vi "Get Panther Dashboard Version.vi"() -> (3 "Panther Dashboard Version":string)   [LabVIEW 2019, in "Panther Dashboard.lvlib"]
uses:
  Panther Dashboard.lvlib
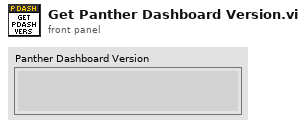
[diagram p1: front panel]
types:
  T1 = cluster{"Major":u16, "Minor":u16, "Fix":u16, "Build":u16}
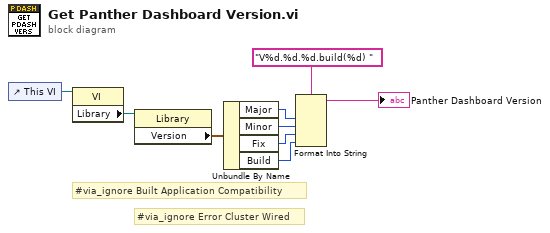
[diagram p0: block diagram]
diagram:
  # "#via_ignore Built Application Compatibility"
  # "#via_ignore Error Cluster Wired"
  n1 = control-ref of="This VI"() -> (w1:refnum<vi>)
  n2 = property class="VI"(reference=w1) -> ("Library"=w3:refnum<vi>)  [unwired: 1 in, 2 out]
  n3 = property class="Library"(reference=w3) -> ("Version"=w4:T1)  [unwired: 1 in, 2 out]
  n4 = Unbundle By Name(w4) -> ("Major"=w5:u16, "Minor"=w6:u16, "Fix"=w7:u16, "Build"=w8:u16)
  n5 = Format Into String(format string="V%d.%d.%d.build(%d) " ("String"), w5, w6, w7, w8) -> (resulting string=→"Panther Dashboard Version":string)  [unwired: 2 in, 1 out]
